vi "Lockin.AppLauncher.vi"() -> ()   [LabVIEW 2019, in "Instrument.Lockin.lvclass"]
uses:
  Instrument.Lockin.lvclass
  <vilib>/JKI/JKI SMO/SMO/Typedefs/SMOState --Enum.ctl
  <vilib>/JKI/JKI SMO/SMO.UI/Typedefs/SMO.UI State--enum.ctl
  C:/Program Files (x86)/National Instruments/LabVIEW 2019/vi.lib/JKI/JKI SMO/SMO/SMO.lvclass
  C:/Program Files (x86)/National Instruments/LabVIEW 2019/user.lib/LevyLab/Instrument Framework/SMOs/Instrument/Instrument.lvclass
  Instrument UI.Lockin/Instrument UI.Lockin.lvclass
  C:/Program Files (x86)/National Instruments/LabVIEW 2019/vi.lib/JKI/JKI SMO/SMO.UI/SMO.UI.lvclass
  C:/Program Files (x86)/National Instruments/LabVIEW 2019/user.lib/LevyLab/Instrument Framework/SMOs/Instrument UI/Instrument UI.lvclass
  <vilib>/JKI/JKI SMO/SMO/SMO.lvclass/SMO.ctl
  <vilib>/JKI/JKI SMO/SMO.UI/SMO.UI.lvclass/SMO.UI.ctl
  <vilib>/numeric/Random Number (Range) U64.vi
  <vilib>/JKI/JKI SMO/SMO/Private/ReftoDVR--SMO.vi
  <vilib>/JKI/JKI SMO/SMO.UI/SMO.UI.ReftoDVR.vi
  <vilib>/numeric/sub_Random U32.vi
  <vilib>/JKI/JKI SMO/SMO/SMO.lvclass
  <vilib>/JKI/JKI SMO/SMO.UI/SMO.UI.lvclass
  <userlib>/LevyLab/Instrument Framework/SMOs/Instrument UI/Instrument UI.lvclass
panel:
  out "error out":errorcluster
  in  "Splash Status":string="Push Start to Start..." caption="String"
  in  "Debug Mode?":bool
  in  "Start":bool=TRUE
  in  "Stop":bool=TRUE
  out "version":string
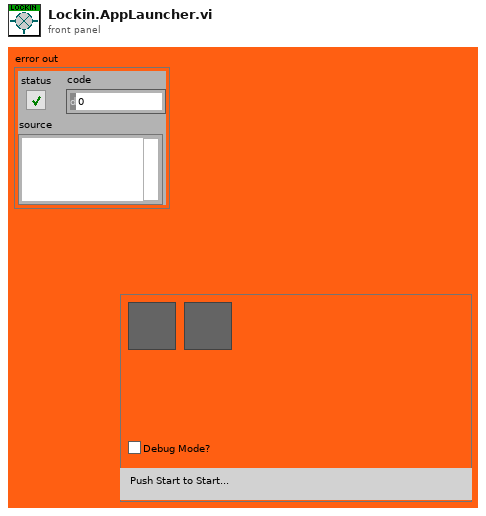
[diagram p1: front panel]
types:
  T1 = typedef "SMO.lvclass/SMOState --Enum.ctl" = enum16{"unknown", "Created", "Started", "Stopped"}
  T2 = typedef "SMO.UI.lvclass/SMO.UI State--enum.ctl" = enum16{"unknown", "Opened", "Closed"}
  T3 = enum32{"Invalid", "Standard", "Closed", "Hidden", "Minimized", "Maximized"}
  T4 = enum32{"invalid app kind", "Development System", "Run Time System", "Student Edition", "Embedded LabVIEW", "Evaluation", "Custom"}
  T5 = cluster{"Core":cluster{"Current VI Reference":refnum<vi>, "Close Panel on Exit?":bool}, "Instrument.Lockin":refnum<class "Instrument.Lockin.lvclass">, "Instrument UI.Lockin":refnum<class "Instrument UI.Lockin.lvclass">}
  T6 = cluster{"Current VI Reference":refnum<vi>, "Close Panel on Exit?":bool}
  T7 = typedef "SMO.lvclass/Public Events.ctl" = cluster{"Error":refnum<user-event>, "State":refnum<user-event>, "Reserve State":refnum<user-event>}
  T8 = typedef "SMO.UI.lvclass/PublicEvents--Cluster.ctl" = cluster{"UI Hidden":refnum<user-event>, "UI State":refnum<user-event>}
  T9 = cluster{"Event Registration Refnum":refnum<event-registration>, "Event Registration Refnum":refnum<event-registration>}
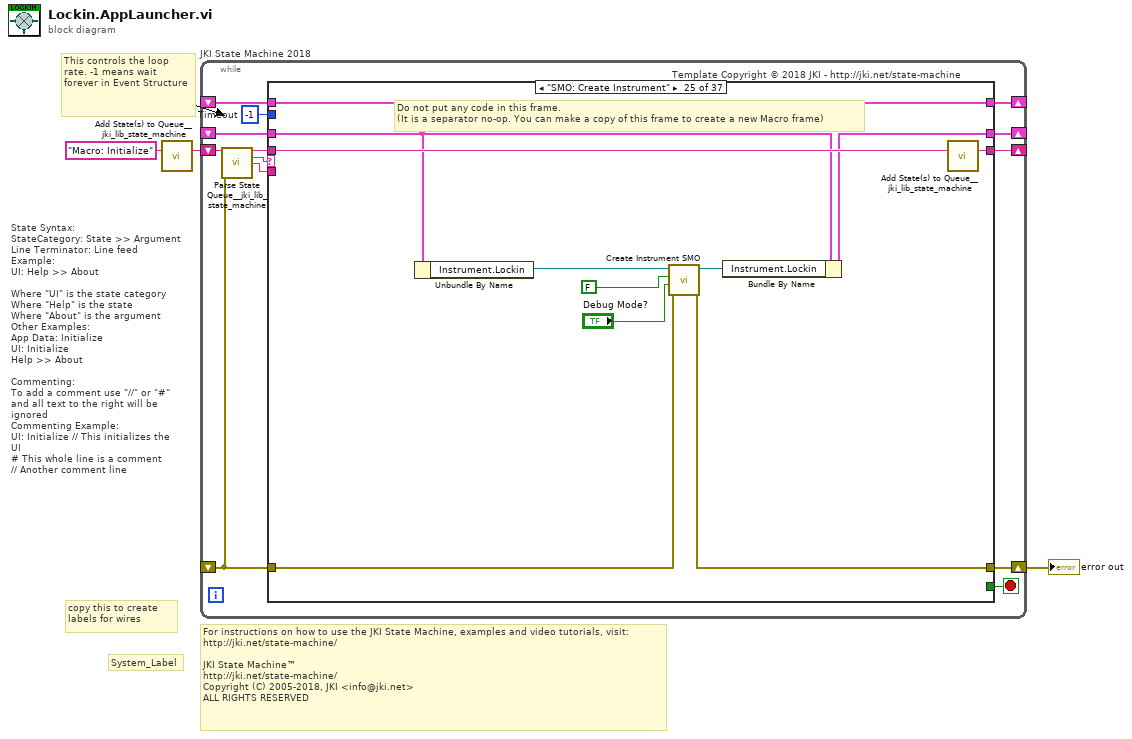
[diagram p0: block diagram]
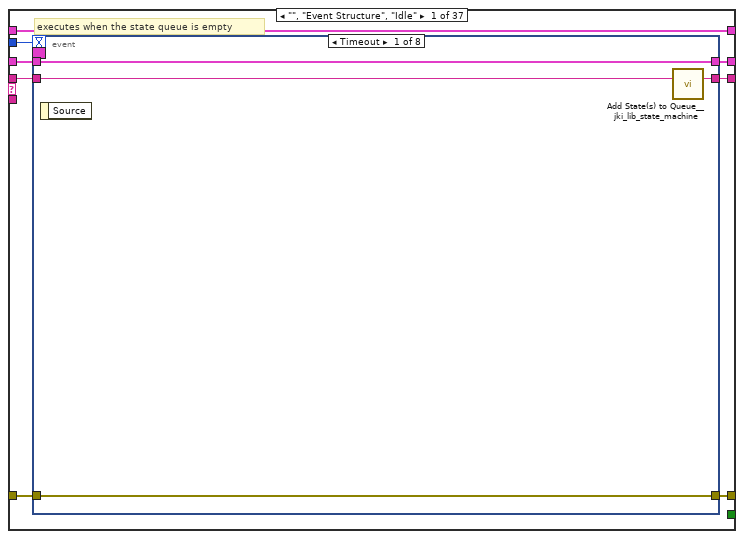
[diagram p2: hidden frame]
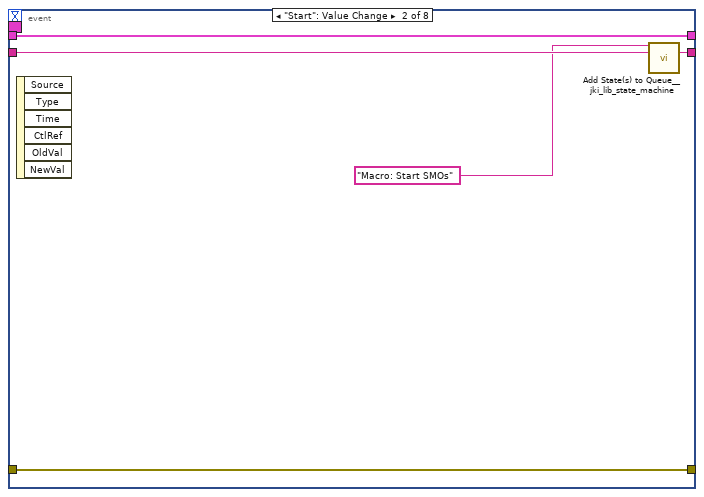
[diagram p3: hidden frame]
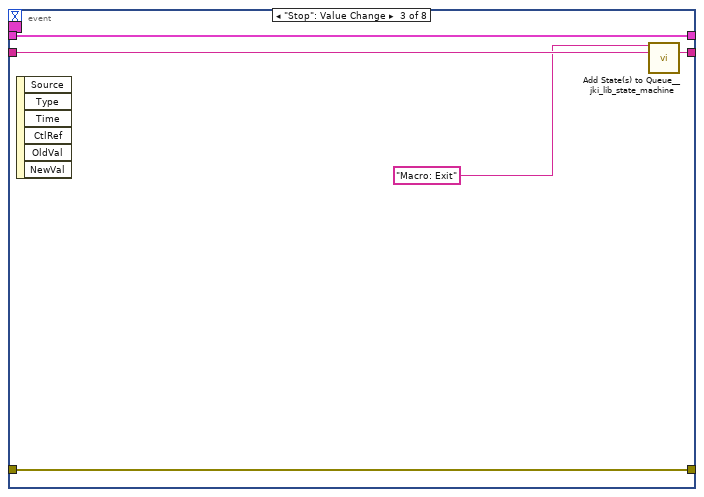
[diagram p4: hidden frame]
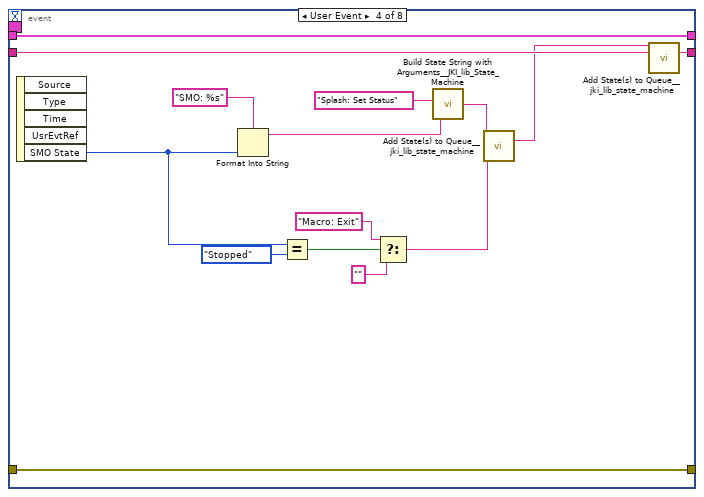
[diagram p5: hidden frame]
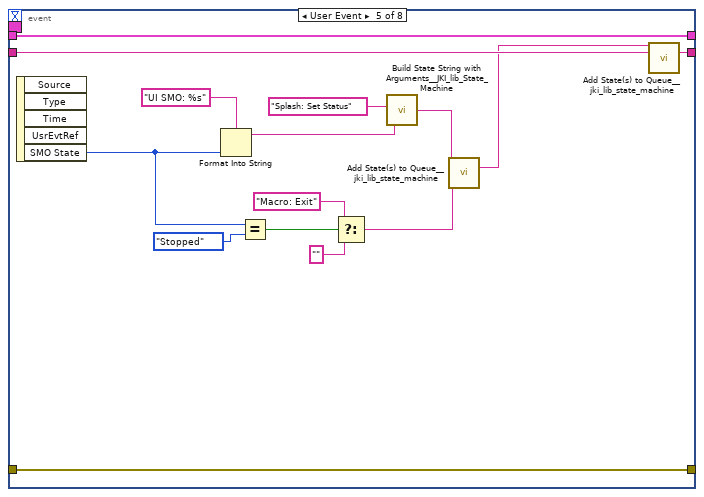
[diagram p6: hidden frame]
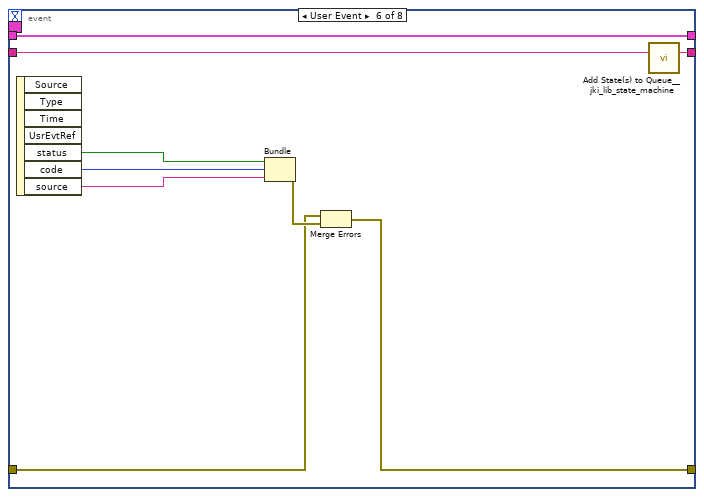
[diagram p7: hidden frame]
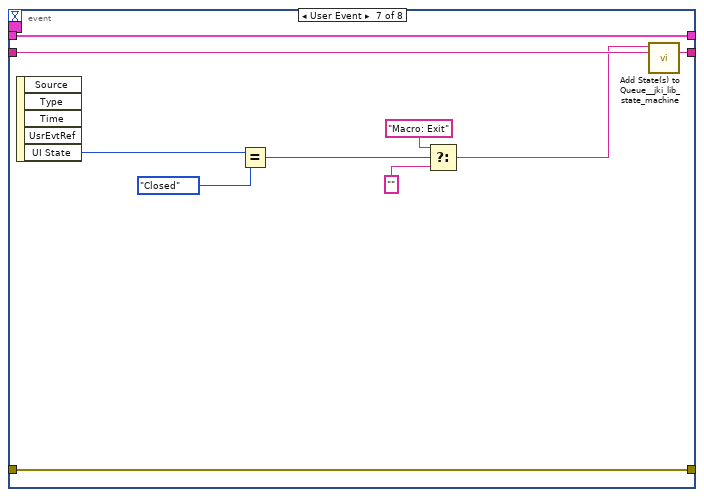
[diagram p8: hidden frame]
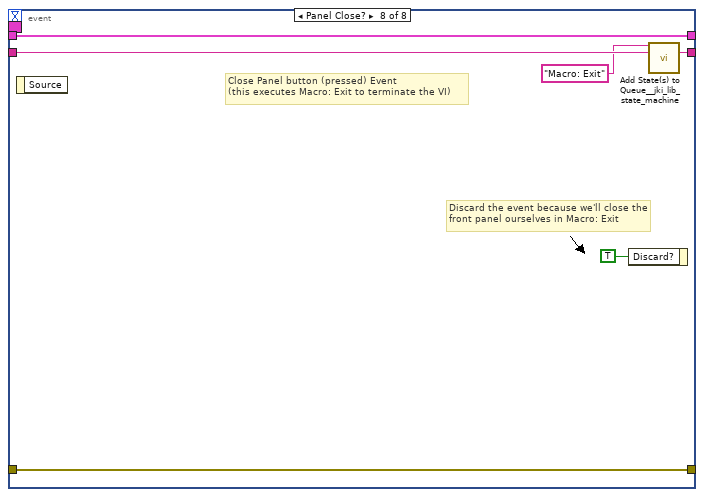
[diagram p9: hidden frame]
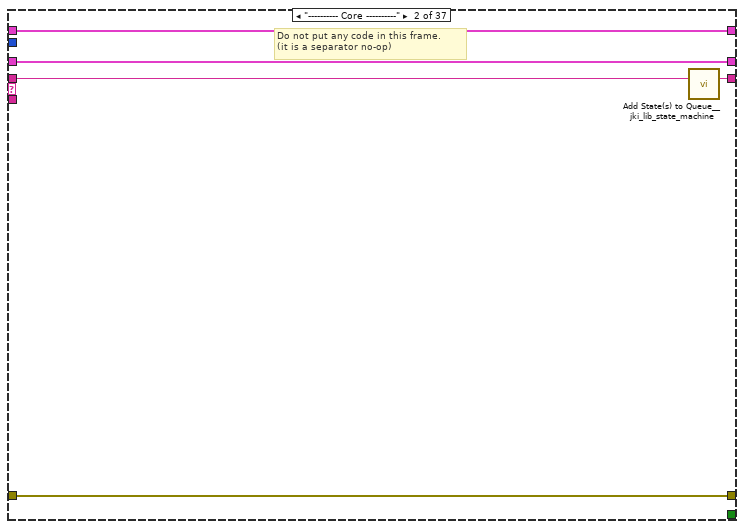
[diagram p10: hidden frame]
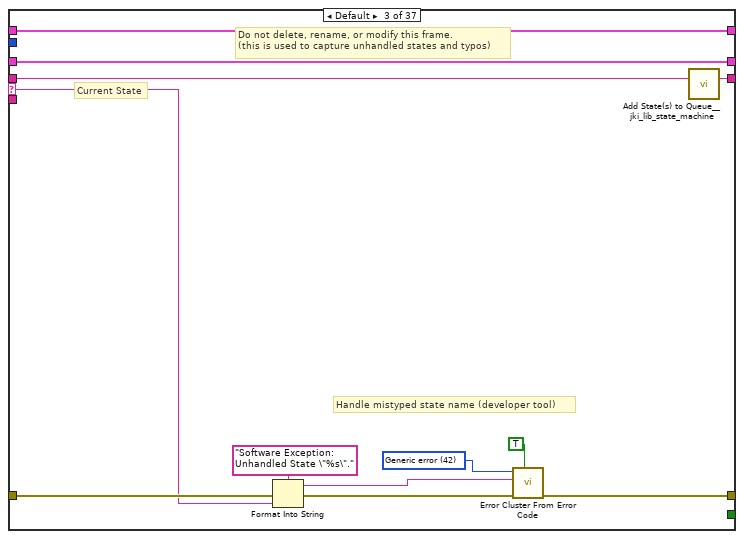
[diagram p11: hidden frame]
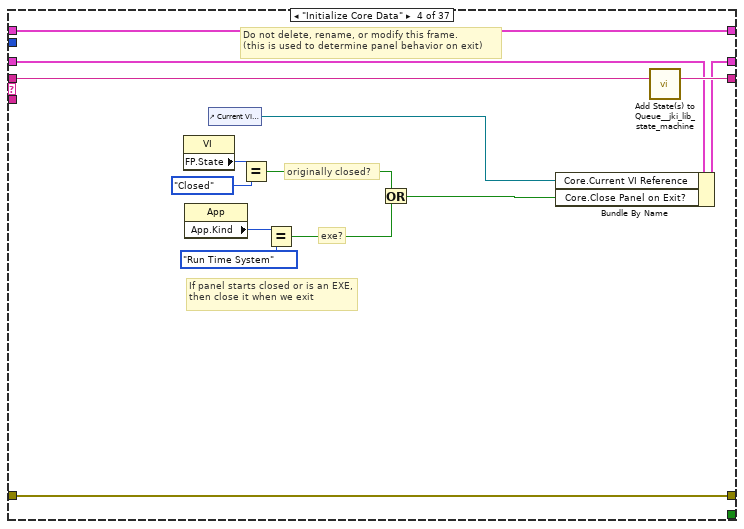
[diagram p12: hidden frame]
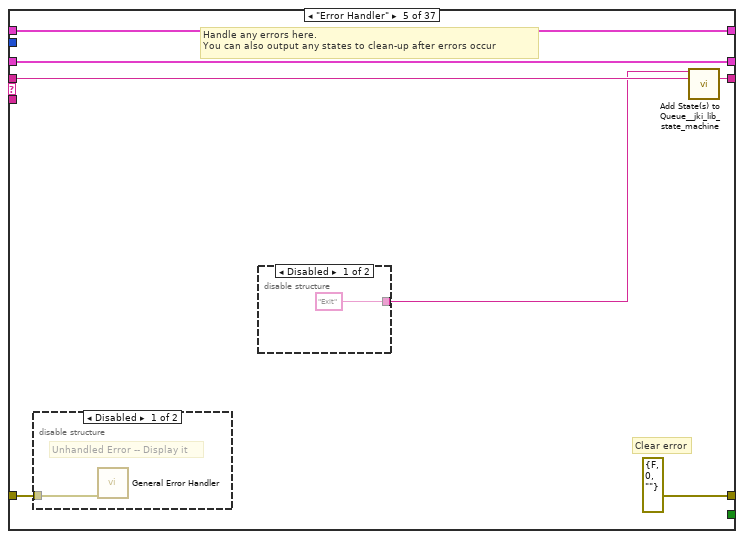
[diagram p13: hidden frame]
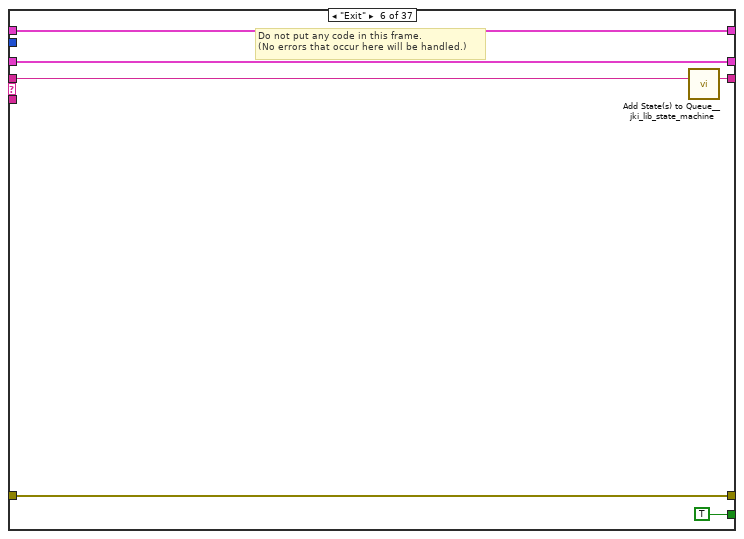
[diagram p16: hidden frame]
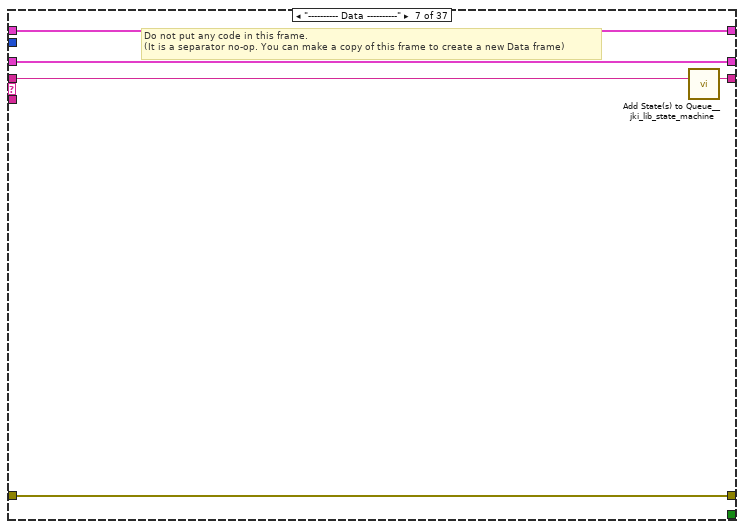
[diagram p17: hidden frame]
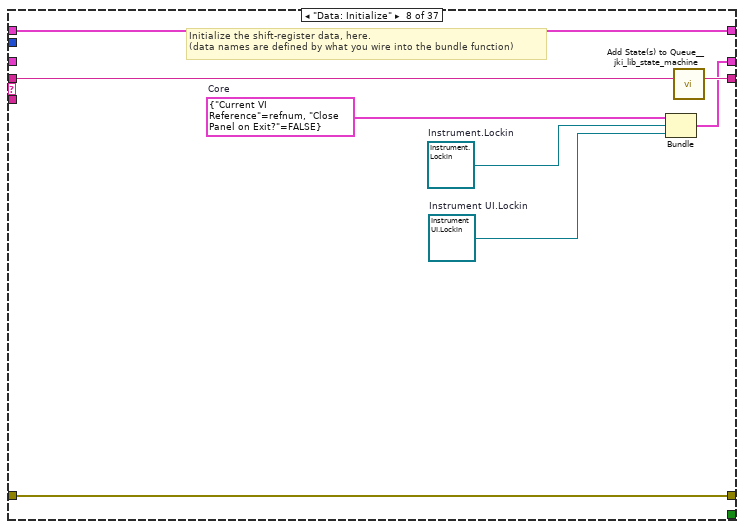
[diagram p18: hidden frame]
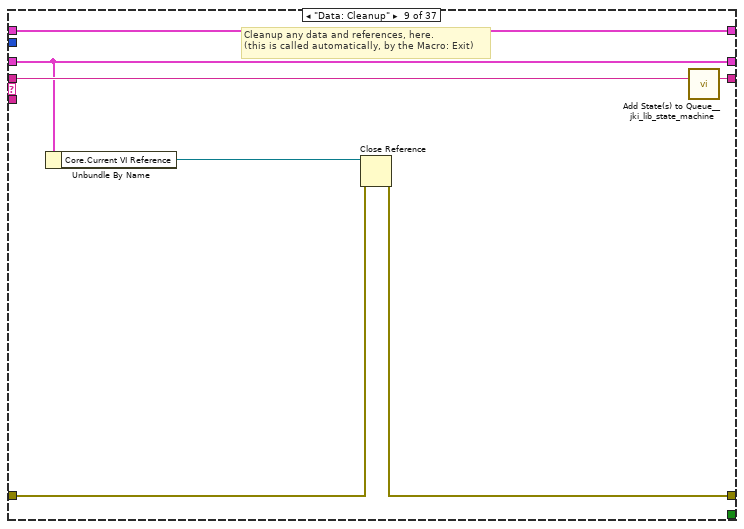
[diagram p19: hidden frame]
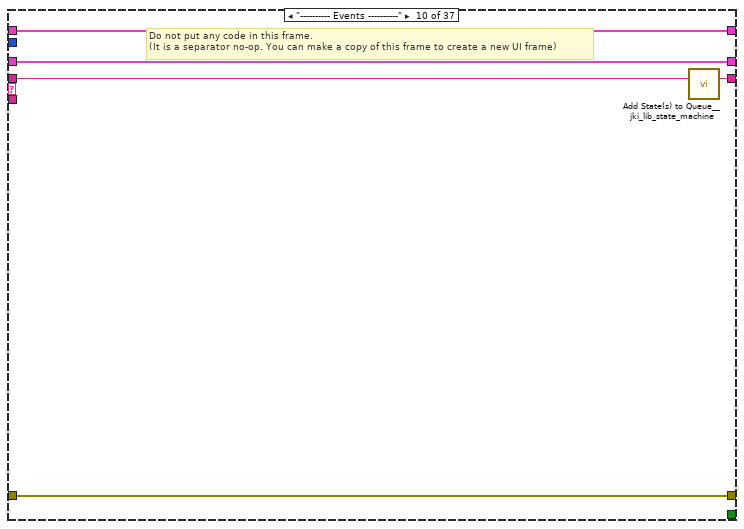
[diagram p20: hidden frame]
diagram:
  # "For instructions on how to use the JKI State Machine, examples and video tutorials, visit:\nhttp://jki.net/state-machine/\n\nJKI State Machine™\nhttp://jki.net/state-machine/\nCopyright (C) 2005-2018, JKI <info@jki.net>\nALL RIGHTS RESERVED"
  # "State Syntax:\nStateCategory: State >> Argument\nLine Terminator: Line feed\nExample:\nUI: Help >> About\n\nWhere \"UI\" is the state category\nWhere \"Help\" is the state\nWhere \"About\" is the argument\nOther Examples:\nApp Data: Initialize\nUI: Initialize\nHelp >> About\n\nCommenting:\nTo add a comment use \"//\" or \"#\" and all text to the right will be ignored\nCommenting Example:\nUI: Initialize // This initializes the UI\n# This whole line is a comment\n// Another comment line"
  # "copy this to create labels for wires"
  # "This controls the loop rate. -1 means wait forever in Event Structure"
  # "System_Label"
  n1 = call <vilib>:"Add State(s) to Queue__jki_lib_state_machine.vi"("State(s) in (\"\")"="Macro: Initialize") -> ("States Out"=w3:string)  [unwired: 14 in]
  n2 = while "JKI State Machine 2018" {
    shift-right: [w9] -> _
    shift-left: _ -> [w4]
    shift-right: [w12] -> w1
    shift-left: _ -> [w7]
    shift-right: [w11] -> _
    shift-left: w3 -> [w13]
    shift-right: [w6] -> _
    shift-left: _ -> [w5]
    stop <- w10 stop-if-true
    w8 = -1  # Timeout
    # "Template Copyright © 2018 JKI - http://jki.net/state-machine"
    n3 = call <vilib>:"Parse State Queue__jki_lib_state_machine.vi"("State Queue"=w13, "Error In (no error)"=w7) -> ("Remaining States"=w15:string, "Current State"=w16:string, "Arguments"=w14:string)  [unwired: 11 in]
    n4 = case shown="\"SMO: Create Instrument\"" w16 {
      selector: w16 -> [_ _ w100 _ _ _ _ _ _ _ _ _ _ _ _ _ _ _ _ _ _ _ _ _ _ _ _ _ _ _ _ _ _ _ _ _ _]
      tunnel: w15 -> [w24 w98 w104 w124 w131 w139 w144 w152 w159 w164 w179 w185 w190 w198 w205 w217 w298 w303 w308 w314 w320 w326 w338 w343 w354 w363 w374 w389 w403 w410 w421 w436 w451 w466 w475 w482 w487]
      tunnel: w14 -> [_ _ _ _ _ _ _ _ _ _ _ _ _ _ w200 w211 _ _ _ _ _ _ _ _ _ _ _ _ _ _ _ _ _ _ _ w479 _]
      tunnel: [w21 w96 w106 w121 errorcluster {"status"=FALSE, "code"=0, "source"=""} ("error out") w136 w142 w149 w155 w162 w168 w180 w188 w193 w201 w214 w289 w301 w306 w312 w318 w324 w336 w341 w347 w355 w371 w385 w397 w404 w417 w432 w448 w463 w473 w477 w485] -> w12
      tunnel: w7 -> [w20 w96 w105 w121 w127 w136 w142 w149 w156 w162 w170 w181 w188 w195 w202 w215 w290 w301 w306 w312 w318 w324 w336 w341 w344 w356 w369 w381 w396 w405 w414 w429 w446 w459 w473 w478 w485]
      tunnel: [w23 w97 w103 w123 w130 w138 w143 w151 w158 w163 w178 w184 w189 w197 w204 w216 w297 w302 w307 w313 w319 w325 w337 w342 w353 w362 w373 w388 w402 w409 w420 w435 w450 w465 w474 w481 w486] -> w11
      tunnel: [_ _ _ _ _ TRUE _ _ _ _ _ _ _ _ _ _ _ _ _ _ _ _ _ _ _ _ _ _ _ _ _ _ _ _ _ _ _] -> w10
      tunnel: [w19 w95 w102 w122 w128 w137 w141 w150 w153 w161 w173 w183 w187 w196 w203 w213 w287 w300 w305 w311 w317 w323 w335 w340 w351 w358 w370 w386 w399 w407 w418 w433 w447 w462 w472 w480 w484] -> w9
      tunnel: w8 -> [w18 _ _ _ _ _ _ _ _ _ _ _ _ _ _ _ _ _ _ _ _ _ _ _ _ _ _ _ _ _ _ _ _ _ _ _ _]
      tunnel: [w17 w94 w99 w111 w125 w134 w140 w147 w154 w160 w176 w182 w186 w194 w199 w210 w288 w299 w304 w309 w316 w322 w329 w339 w352 w361 w372 w387 w401 w408 w419 w434 w449 w464 w471 w476 w483] -> w6
      tunnel: w5 -> [w17 w94 w99 w111 w125 w134 w140 w147 w154 w160 _ w182 w186 w194 w199 w210 w288 w299 w304 w309 w316 w322 w329 w339 w352 w361 w372 w387 w401 w408 w419 w434 w449 w464 w471 w476 w483]
      tunnel: w4 -> [w22 w95 w102 w117 w128 w137 w141 _ w153 w161 w173 w183 w187 w196 w203 w213 w287 w300 w305 w311 w317 w323 w335 w340 w346 w359 w370 w386 w400 w407 w418 w433 w447 w462 w472 w480 w484]
      frame "", "Event Structure", "Idle" {
        # "executes when the state queue is empty"
        n5 = event shown="[0] Timeout" {
          selector: w17 -> [_ _ _ _ _ _ _ _]
          dyn-events: _ -> [_ _ _ _ _ _ _ _]
          timeout: w18 -> [_ _ _ _ _ _ _ _]
          tunnel: w24 -> [w28 w33 w38 w53 w68 w77 w87 w93]
          tunnel: [w27 w32 w37 w52 w67 w76 w86 w92] -> w23
          tunnel: w22 -> [w25 w30 w35 w50 w65 w75 w85 w90]
          tunnel: [w26 w31 w36 w51 w66 w72 w84 w91] -> w21
          tunnel: w20 -> [w26 w31 w36 w51 w66 w73 w84 w91]
          tunnel: [w25 w30 w35 w50 w65 w75 w85 w90] -> w19
          event Timeout {
            n6 = event-data() -> ()  [unwired: 1 in, 1 out]
            n7 = call <vilib>:"Add State(s) to Queue__jki_lib_state_machine.vi"("State(s) in (\"\")"=w28) -> ("States Out"=w27:string)  [unwired: 14 in]
          }
          event "Start": Value Change {
            n8 = event-data() -> ()  [unwired: 1 in, 6 out]
            n9 = call <vilib>:"Add State(s) to Queue__jki_lib_state_machine.vi"("State(s) in Front (\"\")"="Macro: Start SMOs" ("State(s) in Front (\"\")"), "State(s) in (\"\")"=w33) -> ("States Out"=w32:string)  [unwired: 13 in]
          }
          event "Stop": Value Change {
            n10 = event-data() -> ()  [unwired: 1 in, 6 out]
            n11 = call <vilib>:"Add State(s) to Queue__jki_lib_state_machine.vi"("State(s) in Front (\"\")"="Macro: Exit" ("State(s) in Front (\"\")"), "State(s) in (\"\")"=w38) -> ("States Out"=w37:string)  [unwired: 13 in]
          }
          event User Event {
            n12 = event-data() -> ("SMO State"=w45:T1)  [unwired: 1 in, 4 out]
            n13 = Format Into String(format string="SMO: %s", w45) -> (resulting string=w42:string)  [unwired: 2 in, 1 out]
            n14 = Equal?(x=w45, y=SMOState_--Enum."Stopped") -> (x = y?=w48:bool)
            n15 = Select(t="Macro: Exit", s=w48, f="" ("State(s) in Front (\"\")")) -> (s? t:f=w40:string)
            n16 = call <vilib>:"Build State String with Arguments__JKI_lib_State_Machine.vi"("Arguments (\"\")"=w42, "State"="Splash: Set Status" ("t")) -> ("State with Arguments"=w41:string)  [unwired: 4 in]
            n17 = call <vilib>:"Add State(s) to Queue__jki_lib_state_machine.vi"("State(s) in Front (\"\")"=w41, "State(s) at Back (\"\")"=w40) -> ("States Out"=w39:string)  [unwired: 13 in]
            n18 = call <vilib>:"Add State(s) to Queue__jki_lib_state_machine.vi"("State(s) in Front (\"\")"=w39, "State(s) in (\"\")"=w53) -> ("States Out"=w52:string)  [unwired: 13 in]
          }
          event User Event {
            n19 = event-data() -> ("SMO State"=w56:T1)  [unwired: 1 in, 4 out]
            n20 = Format Into String(format string="UI SMO: %s", w56) -> (resulting string=w60:string)  [unwired: 2 in, 1 out]
            n21 = Equal?(x=w56, y=SMOState_--Enum."Stopped") -> (x = y?=w64:bool)
            n22 = Select(t="Macro: Exit", s=w64, f="" ("State(s) in Front (\"\")")) -> (s? t:f=w59:string)
            n23 = call <vilib>:"Build State String with Arguments__JKI_lib_State_Machine.vi"("Arguments (\"\")"=w60, "State"="Splash: Set Status" ("t")) -> ("State with Arguments"=w57:string)  [unwired: 4 in]
            n24 = call <vilib>:"Add State(s) to Queue__jki_lib_state_machine.vi"("State(s) in Front (\"\")"=w57, "State(s) at Back (\"\")"=w59) -> ("States Out"=w58:string)  [unwired: 13 in]
            n25 = call <vilib>:"Add State(s) to Queue__jki_lib_state_machine.vi"("State(s) in Front (\"\")"=w58, "State(s) in (\"\")"=w68) -> ("States Out"=w67:string)  [unwired: 13 in]
          }
          event User Event {
            n26 = event-data() -> ("status"=w69:bool, "code"=w71:i32, "source"=w70:string)  [unwired: 1 in, 4 out]
            n27 = Bundle("status"=w69, "code"=w71, "source"=w70) -> (w74:errorcluster)  [unwired: 1 in]
            n28 = Merge Errors(w73, w74) -> (w72:errorcluster)
            n29 = call <vilib>:"Add State(s) to Queue__jki_lib_state_machine.vi"("State(s) in (\"\")"=w77) -> ("States Out"=w76:string)  [unwired: 14 in]
          }
          event User Event {
            n30 = event-data() -> ("UI State"=w83:T2)  [unwired: 1 in, 4 out]
            n31 = Equal?(x=w83, y=SMO.UI_State--enum."Closed" ("UI State")) -> (x = y?=w81:bool)
            n32 = Select(t="Macro: Exit", s=w81, f="") -> (s? t:f=w78:string)
            n33 = call <vilib>:"Add State(s) to Queue__jki_lib_state_machine.vi"("State(s) in Front (\"\")"=w78, "State(s) in (\"\")"=w87) -> ("States Out"=w86:string)  [unwired: 13 in]
          }
          event Panel Close? {
            # "Discard the event because we'll close the front panel ourselves in Macro: Exit"
            # "Close Panel button (pressed) Event\n(this executes Macro: Exit to terminate the VI)"
            n34 = event-data() -> ()  [unwired: 1 in, 1 out]
            n35 = event-data("Discard?"=TRUE) -> ()  [unwired: 1 in, 1 out]
            n36 = call <vilib>:"Add State(s) to Queue__jki_lib_state_machine.vi"("State(s) in Front (\"\")"="Macro: Exit", "State(s) in (\"\")"=w93) -> ("States Out"=w92:string)  [unwired: 13 in]
          }
        }
      }
      frame "---------- Core ----------" {
        # "Do not put any code in this frame.\n(it is a separator no-op)"
        n37 = call <vilib>:"Add State(s) to Queue__jki_lib_state_machine.vi"("State(s) in (\"\")"=w98) -> ("States Out"=w97:string)  [unwired: 14 in]
      }
      frame Default {
        w109 = 42 items=["No error", "Argument error", "Memory is full", "Out of zone", "End of file", "File already open", "Generic file I/O error", "File not found", "File permission error", "Disk is full", "Duplicate path", "Too many files open", "System feature not enabled", "Resource file not found", "Cannot add resource", "Resource not found", "Image not found", "Image memory error", "Pen does not exist", "Config type invalid", "Config token not found", "Config parse error", "Config memory error", "Bad external code format", "Bad external code offset", "External code not present", "Null window", "Destroy window error", "Null menu", "Print aborted", "Bad print record", "Print driver error", "Windows error during printing", "Memory error during printing", "Print dialog error", "Generic print error", "Invalid device refnum", "Device not found", "Device parameter error", "Device unit error", "Cannot open device", "Device call aborted", "Generic error", "Cancelled by user", "Object ID too low", "Object ID too high", "Object not in heap", "Unknown heap", "Unknown object (invalid DefProc)", "Unknown object (DefProc not in table)", "Message out of range", "Invalid (null) method", "Unknown message", "Manager call not supported", "Bad address", "Network operation in progress", "Network operation timed out", "Connection is busy", "Network attribute not supported", "Network error", "Address in use", "System out of memory", "Connection aborted", "Connection refused", "Not connected", "Already connected", "Connection closed", "Initialization error (interapplication manager)", "Bad occurrence", "Wait on unbound occurrence handler", "Occurrence queue overflow", "Datalog type conflict", "Unused", "Unrecognized type (interapplication manager)", "Memory corrupt", "Failed to make temporary DLL", "Old CIN version", "Drag socket not found", "Failed to load drop-object", "Failed to register OLE object", "Failed to release OLE object", "Format specifier type mismatch", "Unknown format specifier", "Too few format specifiers", "Too many format specifiers", "Scan failed", "Newer CIN version", "Error converting to variant", "Runtime menu error", "Password tampered", "Variant attribute not found", "Incompatible variant data type", "Event data is not available", "Event Store is not present", "Occurrence is not found", "Event Queue is not created", "Event info is not available", "Refnum passed is NULL", "Error retrieving Class GUID", "Error retrieving CoClass GUID", "Error retrieving TypeLib GUID.", "Bad built application magic bytes.", "Specific driver is different from the specific driver associated with the Logical Name.", "There is no session opened to the class driver.", "Max Error", "MAX - Error with config objects", "MAX - Error loading configuration", "MAX - Group not supported"]
        # "Current State"
        # "Do not delete, rename, or modify this frame.\n(this is used to capture unhandled states and typos)"
        # "Handle mistyped state name (developer tool)"
        n38 = Format Into String(format string="Software Exception: Unhandled State \"%s\"." ("message"), error in=w105, w100) -> (resulting string=w108:string, error out=w107:errorcluster)  [unwired: 1 in]
        n39 = call <vilib>:"Error Cluster From Error Code.vi"("show call chain? (False)"=TRUE, "error in (no error)"=w107, "error message (\"\")"=w108, "error code (0)"=w109) -> ("error out"=w106:errorcluster)  [unwired: 5 in]
        n40 = call <vilib>:"Add State(s) to Queue__jki_lib_state_machine.vi"("State(s) in (\"\")"=w104) -> ("States Out"=w103:string)  [unwired: 14 in]
      }
      frame "Initialize Core Data" {
        # "Do not delete, rename, or modify this frame.\n(this is used to determine panel behavior on exit)"
        # "originally closed?"
        # "exe?"
        # "If panel starts closed or is an EXE, then close it when we exit"
        n41 = property class="VI"() -> ("FP.State"=w114:T3)  [unwired: 2 in, 2 out]
        n42 = property class="App"() -> ("App.Kind"=w120:T4)  [unwired: 2 in, 2 out]
        n43 = control-ref of="Current VI Reference"() -> (w115:refnum<vi>)
        n44 = Equal?(x=w114, y=T3."Closed" ("Front Panel Window:State")) -> (x = y?=w112:bool)
        n45 = Equal?(x=w120, y=T4."Run Time System" ("Application:Kind")) -> (x = y?=w118:bool)
        n46 = Or(x=w112, y=w118) -> (x .or. y?=w116:bool)
        n47 = Bundle By Name(cluster=w117, "Core.Current VI Reference"=w115, "Core.Close Panel on Exit?"=w116) -> (w122:T5)
        n48 = call <vilib>:"Add State(s) to Queue__jki_lib_state_machine.vi"("State(s) in (\"\")"=w124) -> ("States Out"=w123:string)  [unwired: 14 in]
      }
      frame "Error Handler" {
        # "Handle any errors here.\nYou can also output any states to clean-up after errors occur"
        # "Clear error"
        n49 = disable-structure shown="Disabled" {
          disable-tunnel: w127 -> [w133 _]
          frame Disabled {
            # "Unhandled Error -- Display it"
            n50 = call <vilib>:"General Error Handler.vi"("error in (no error)"=w133) -> ()  [unwired: 10 in, 5 out]
          }
          frame Enabled {
          }
        }
        n51 = disable-structure shown="Disabled" {
          disable-tunnel: ["Exit" _] -> w126
          frame Disabled {
          }
          frame Enabled {
          }
        }
        n52 = call <vilib>:"Add State(s) to Queue__jki_lib_state_machine.vi"("State(s) in Front (\"\")"=w126, "State(s) in (\"\")"=w131) -> ("States Out"=w130:string)  [unwired: 13 in]
      }
      frame "Exit" {
        # "Do not put any code in this frame.\n(No errors that occur here will be handled.)"
        n53 = call <vilib>:"Add State(s) to Queue__jki_lib_state_machine.vi"("State(s) in (\"\")"=w139) -> ("States Out"=w138:string)  [unwired: 14 in]
      }
      frame "---------- Data ----------" {
        # "Do not put any code in this frame.\n(It is a separator no-op. You can make a copy of this frame to create a new Data frame)"
        n54 = call <vilib>:"Add State(s) to Queue__jki_lib_state_machine.vi"("State(s) in (\"\")"=w144) -> ("States Out"=w143:string)  [unwired: 14 in]
      }
      frame "Data: Initialize" {
        w146 = refnum<class "Instrument UI.Lockin.lvclass"> refnum  # Instrument UI.Lockin
        w145 = refnum<class "Instrument.Lockin.lvclass"> refnum  # Instrument.Lockin
        w148 = T6 {"Current VI Reference"=refnum, "Close Panel on Exit?"=FALSE}  # Core
        # "Initialize the shift-register data, here.\n(data names are defined by what you wire into the bundle function)"
        n55 = Bundle("Core"=w148, "Instrument.Lockin"=w145, "Instrument UI.Lockin"=w146) -> (w150:T5)  [unwired: 1 in]
        n56 = call <vilib>:"Add State(s) to Queue__jki_lib_state_machine.vi"("State(s) in (\"\")"=w152) -> ("States Out"=w151:string)  [unwired: 14 in]
      }
      frame "Data: Cleanup" {
        # "Cleanup any data and references, here.\n(this is called automatically, by the Macro: Exit)"
        n57 = Unbundle By Name(w153) -> ("Core.Current VI Reference"=w157:refnum<vi>)
        n58 = Close Reference(reference=w157, error in (no error)=w156) -> (error out=w155:errorcluster)
        n59 = call <vilib>:"Add State(s) to Queue__jki_lib_state_machine.vi"("State(s) in (\"\")"=w159) -> ("States Out"=w158:string)  [unwired: 14 in]
      }
      frame "---------- Events ----------" {
        # "Do not put any code in this frame.\n(It is a separator no-op. You can make a copy of this frame to create a new UI frame)"
        n60 = call <vilib>:"Add State(s) to Queue__jki_lib_state_machine.vi"("State(s) in (\"\")"=w164) -> ("States Out"=w163:string)  [unwired: 14 in]
      }
      frame "Events: Register" {
        # "Do not put any code in this frame.\n(It is a separator no-op. You can make a copy of this frame to create a new UI frame)"
        n61 = Unbundle By Name(w173) -> ("Instrument.Lockin"=w172:refnum<class "Instrument.Lockin.lvclass">, "Instrument UI.Lockin"=w171:refnum<class "Instrument UI.Lockin.lvclass">)
        n62 = call <vilib>:"GetPublicEvents.vi"("error in (no error)"=w170, "SMO"=w172) -> ("error out"=w169:errorcluster, "Public Events"=w174:T7)  [unwired: 7 in, 1 out]
        n63 = call <vilib>:"GetPublicEvents.vi"("error in (no error)"=w169, "SMO"=w171) -> ("error out"=w168:errorcluster, "Public Events"=w175:T7, "SMO out"=w166:refnum<class "Instrument UI.Lockin.lvclass">)  [unwired: 7 in]
        n64 = register-events(w174) -> (reference out=w177:refnum<event-registration>)  [unwired: 2 in, 1 out]
        n65 = call <vilib>:"SMO.UI.GetPublicEvents.vi"("SMO.UI"=w166) -> ("SMO.UI Public Events"=w165:T8)  [unwired: 8 in, 2 out]
        n66 = register-events(w175, w165) -> (reference out=w167:refnum<event-registration>)  [unwired: 2 in, 1 out]
        n67 = Bundle("Event Registration Refnum"=w177, "Event Registration Refnum"=w167) -> (w176:T9)  [unwired: 1 in]
        n68 = call <vilib>:"Add State(s) to Queue__jki_lib_state_machine.vi"("State(s) in (\"\")"=w179) -> ("States Out"=w178:string)  [unwired: 14 in]
      }
      frame "Events: Unregister" {
        # "Do not put any code in this frame.\n(It is a separator no-op. You can make a copy of this frame to create a new UI frame)"
        n69 = Unregister For Events(event registration refnum=w182, error in=w181) -> (error out=w180:errorcluster)
        n70 = call <vilib>:"Add State(s) to Queue__jki_lib_state_machine.vi"("State(s) in (\"\")"=w185) -> ("States Out"=w184:string)  [unwired: 14 in]
      }
      frame "---------- UI ----------" {
        # "Do not put any code in this frame.\n(It is a separator no-op. You can make a copy of this frame to create a new UI frame)"
        n71 = call <vilib>:"Add State(s) to Queue__jki_lib_state_machine.vi"("State(s) in (\"\")"=w190) -> ("States Out"=w189:string)  [unwired: 14 in]
      }
      frame "UI: Initialize" {
        # "Initialize the User Interface, here.\n(this is called automatically, by the Macro: Init)"
        n72 = invoke on="Start" class="Bool (strict)" method="Reinit To Default"() -> ()  [unwired: 3 in, 3 out]
        n73 = invoke on="Stop" class="Bool (strict)" method="Reinit To Default"() -> ()  [unwired: 3 in, 3 out]
        n74 = invoke on="error out" class="Clust (strict)" method="Reinit To Default"() -> ()  [unwired: 3 in, 3 out]
        n75 = call <userlib>:"Fit VI window to Largest Dec__ogtk.vi"("error in (no error)"=w195, "border spacing (2 px)"=-1) -> ("error out"=w193:errorcluster)  [unwired: 4 in, 1 out]
        n76 = call <userlib>:"MGI Get Executable Version.vi"() -> ("Version"=→"version":string)  [unwired: 7 in]
        n77 = call <vilib>:"Add State(s) to Queue__jki_lib_state_machine.vi"("State(s) in (\"\")"=w198) -> ("States Out"=w197:string)  [unwired: 14 in]
      }
      frame "UI: Cursor Set" {
        # "Argument"
        # "Set and Unset Cursor Busy.\n(Usage: \"UI: Cursor Set >> Busy|Idle\")"
        n78 = case shown="\"Busy\"" w200 {
          tunnel: w202 -> [w207 w209]
          tunnel: [w206 w208] -> w201
          frame "Idle", Default {
            n79 = call <vilib>:"Unset Busy.vi"("error in (no error)"=w207) -> ("error out"=w206:errorcluster)  [unwired: 10 in]
          }
          frame "Busy" {
            n80 = call <vilib>:"Set Busy.vi"("error in (no error)"=w209) -> ("error out"=w208:errorcluster)  [unwired: 9 in, 1 out]
          }
        }
        n81 = call <vilib>:"Add State(s) to Queue__jki_lib_state_machine.vi"("State(s) in (\"\")"=w205) -> ("States Out"=w204:string)  [unwired: 14 in]
      }
      frame "UI: Front Panel State" {
        # "Argument"
        # "Set Front Panel Open or Closed\n(Usage: \"UI: Front Panel State >> Open|Close\")"
        n82 = Unbundle By Name(w213) -> ("Core.Current VI Reference"=w212:refnum<vi>)
        n83 = case shown="\"Open\", \"Standard\", Default" w211 {
          tunnel: w215 -> [w223 w238 w249 w262 w275]
          tunnel: [w225 w239 w251 w264 w277] -> w214
          tunnel: w212 -> [w224 w236 w250 w263 w276]
          frame "Open", "Standard", Default {
            w218 = T3."Standard" ("State")
            n84 = property class="VI"(reference=w224, error in=w223) -> (reference out=w221:refnum<vi>, error out=w222:errorcluster, "FP.State"=w220:T3)
            n85 = Not Equal?(x=w220, y=w218) -> (x != y?=w219:bool)
            n86 = case shown="False" w219 {
              tunnel: [w229 w231] -> w225
              tunnel: w222 -> [w228 w231]
              tunnel: w221 -> [w227 _]
              tunnel: w218 -> [w226 _]
              frame True {
                n87 = invoke class="VI" method="FP.Open"(reference=w227, error in=w228, "Activate"=TRUE, "State"=w226) -> (error out=w229:errorcluster)  [unwired: 1 in, 4 out]
              }
              frame False {
              }
            }
          }
          frame "Close", "Closed" {
            n88 = property class="VI"(reference=w236, error in=w238) -> (reference out=w235:refnum<vi>, error out=w237:errorcluster, "FP.State"=w233:T3)
            n89 = Not Equal?(x=w233, y=T3."Closed" ("Front Panel Window:State")) -> (x != y?=w232:bool)
            n90 = case shown="True" w232 {
              tunnel: [w240 w243] -> w239
              tunnel: w237 -> [w240 w242]
              tunnel: w235 -> [_ w241]
              frame False {
              }
              frame True {
                n91 = invoke class="VI" method="FP.Close"(reference=w241, error in=w242) -> (error out=w243:errorcluster)  [unwired: 1 in, 2 out]
              }
            }
          }
          frame "Hidden", "Hide" {
            w244 = T3."Hidden" ("State")
            n92 = property class="VI"(reference=w250, error in=w249) -> (reference out=w247:refnum<vi>, error out=w248:errorcluster, "FP.State"=w246:T3)
            n93 = Not Equal?(x=w246, y=w244) -> (x != y?=w245:bool)
            n94 = case shown="True" w245 {
              tunnel: [w255 w256] -> w251
              tunnel: w248 -> [w254 w256]
              tunnel: w247 -> [w253 _]
              tunnel: w244 -> [w252 _]
              frame True {
                n95 = invoke class="VI" method="FP.Open"(reference=w253, error in=w254, "State"=w252) -> (error out=w255:errorcluster)  [unwired: 2 in, 4 out]
              }
              frame False {
              }
            }
          }
          frame "Minimize", "Minimized" {
            w257 = T3."Minimized" ("State")
            n96 = property class="VI"(reference=w263, error in=w262) -> (reference out=w260:refnum<vi>, error out=w261:errorcluster, "FP.State"=w259:T3)
            n97 = Not Equal?(x=w259, y=w257) -> (x != y?=w258:bool)
            n98 = case shown="True" w258 {
              tunnel: [w268 w269] -> w264
              tunnel: w261 -> [w267 w269]
              tunnel: w260 -> [w266 _]
              tunnel: w257 -> [w265 _]
              frame True {
                n99 = invoke class="VI" method="FP.Open"(reference=w266, error in=w267, "State"=w265) -> (error out=w268:errorcluster)  [unwired: 2 in, 4 out]
              }
              frame False {
              }
            }
          }
          frame "Maximize", "Maximized" {
            w270 = T3."Maximized" ("State")
            n100 = property class="VI"(reference=w276, error in=w275) -> (reference out=w273:refnum<vi>, error out=w274:errorcluster, "FP.State"=w272:T3)
            n101 = Not Equal?(x=w272, y=w270) -> (x != y?=w271:bool)
            n102 = case shown="True" w271 {
              tunnel: [w281 w282] -> w277
              tunnel: w274 -> [w280 w282]
              tunnel: w273 -> [w279 _]
              tunnel: w270 -> [w278 _]
              frame True {
                n103 = invoke class="VI" method="FP.Open"(reference=w279, error in=w280, "State"=w278) -> (error out=w281:errorcluster)  [unwired: 2 in, 4 out]
              }
              frame False {
              }
            }
          }
        }
        n104 = call <vilib>:"Add State(s) to Queue__jki_lib_state_machine.vi"("State(s) in (\"\")"=w217) -> ("States Out"=w216:string)  [unwired: 14 in]
      }
      frame "UI: Set Background Color" {
        # "Do not put any code in this frame.\n(It is a separator no-op. You can make a copy of this frame to create a new UI frame)"
        n105 = property class="VI"(error in=w290) -> (error out=w292:errorcluster, "Panel"=w293:refnum<vi>)  [unwired: 1 in, 1 out]
        n106 = property class="Pnl"(reference=w293, error in=w292) -> (error out=w291:errorcluster, "Panes[]"=w294:refnum<vi>[])  [unwired: 1 out]
        n107 = call-poly <vilib>:"Random Number (Range).vi"("lower bound (0)"=u32 16736018 ("Color Box"), "upper bound (100)"=u32 16711708 ("Color Box")) -> ("number"=w284:u64)  [unwired: 9 in]
        n108 = Index Array(array=w294, index=0) -> (element=w296:refnum<vi>)
        n109 = To Unsigned Long Integer(number=w284) -> (unsigned 32bit integer=w283:u32)
        n110 = property class="Pane"(reference=w296, error in=w291, "PaneColor"=w283) -> (error out=w289:errorcluster)  [unwired: 1 out]
        n111 = call <vilib>:"Add State(s) to Queue__jki_lib_state_machine.vi"("State(s) in (\"\")"=w298) -> ("States Out"=w297:string)  [unwired: 14 in]
      }
      frame "UI: Exit" {
        # "Do not put any code in this frame.\n(It is a separator no-op. You can make a copy of this frame to create a new UI frame)"
        n112 = invoke on="Start" class="Bool (strict)" method="Reinit To Default"() -> ()  [unwired: 3 in, 3 out]
        n113 = invoke on="Stop" class="Bool (strict)" method="Reinit To Default"() -> ()  [unwired: 3 in, 3 out]
        n114 = call <vilib>:"Add State(s) to Queue__jki_lib_state_machine.vi"("State(s) in (\"\")"=w303) -> ("States Out"=w302:string)  [unwired: 14 in]
      }
      frame "---------- Macro ----------" {
        # "Do not put any code in this frame.\n(It is a separator no-op. You can make a copy of this frame to create a new Macro frame)"
        n115 = call <vilib>:"Add State(s) to Queue__jki_lib_state_machine.vi"("State(s) in (\"\")"=w308) -> ("States Out"=w307:string)  [unwired: 14 in]
      }
      frame "Macro: Initialize" {
        # "Initialization Macro\n(This is called once, when the VI starts)"
        n116 = call <vilib>:"Add State(s) to Queue__jki_lib_state_machine.vi"("State(s) in Front (\"\")"="Data: Initialize\nInitialize Core Data\n//Events: Register\nUI: Initialize\nUI: Front Panel State >> Open\nUI: Set Background Color\nSplash: Set Status >> Push Start to Start...", "State(s) in (\"\")"=w314) -> ("States Out"=w313:string)  [unwired: 13 in]
      }
      frame "Macro: Start SMOs" {
        # "Do not put any code in this frame.\n(It is a separator no-op. You can make a copy of this frame to create a new Macro frame)"
        n117 = call <vilib>:"Add State(s) to Queue__jki_lib_state_machine.vi"("State(s) in Front (\"\")"="Splash: Set Status >> Starting Instrument...\nSMO: Create Instrument\nSMO: Create Instrument UI\nEvents: Register\nSMO: Start Instrument\nSplash: Set Status >> Instrument Process Started...\nSplash: Set Status >> Starting User Interface...\nSMO: Start Instrument UI\nUI: Front Panel State >> Hide\nSMO: Show Instrument UI" ("State(s) in Front (\"\")"), "State(s) in (\"\")"=w320) -> ("States Out"=w319:string)  [unwired: 13 in]
      }
      frame "Macro: Stop SMOs" {
        # "Do not put any code in this frame.\n(It is a separator no-op. You can make a copy of this frame to create a new Macro frame)"
        n118 = call <vilib>:"Add State(s) to Queue__jki_lib_state_machine.vi"("State(s) in Front (\"\")"="//SMO: Hide Instrument UI\nSMO: Stop Instrument UI\nSMO: Stop Instrument\nSMO: Destroy Instrument UI\nSMO: Destroy Instrument" ("State(s) in Front (\"\")"), "State(s) in (\"\")"=w326) -> ("States Out"=w325:string)  [unwired: 13 in]
      }
      frame "Macro: Exit" {
        # "Exit Macro\n(This is called once, when the VI exits)"
        n119 = Unbundle By Name(w335) -> ("Core.Close Panel on Exit?"=w334:bool)
        n120 = Select(t="UI: Front Panel State >> Open", s=w334, f="") -> (s? t:f=w331:string)
        n121 = call <vilib>:"Add State(s) to Queue__jki_lib_state_machine.vi"("State(s) in Front (\"\")"="UI: Front Panel State >> Open\nUI: Exit", "State(s) in (\"\")"=w331, "State(s) at Back (\"\")"="Macro: Stop SMOs\nData: Cleanup\nEvents: Unregister\nExit") -> ("States Out"=w330:string)  [unwired: 12 in]
        n122 = call <vilib>:"Add State(s) to Queue__jki_lib_state_machine.vi"("State(s) in Front (\"\")"=w330, "State(s) in (\"\")"=w338) -> ("States Out"=w337:string)  [unwired: 13 in]
      }
      frame "---------- SMO ----------" {
        # "Do not put any code in this frame.\n(It is a separator no-op. You can make a copy of this frame to create a new Macro frame)"
        n123 = call <vilib>:"Add State(s) to Queue__jki_lib_state_machine.vi"("State(s) in (\"\")"=w343) -> ("States Out"=w342:string)  [unwired: 14 in]
      }
      frame "SMO: Create Instrument" {
        # "Do not put any code in this frame.\n(It is a separator no-op. You can make a copy of this frame to create a new Macro frame)"
        n124 = Unbundle By Name(w346) -> ("Instrument.Lockin"=w345:refnum<class "Instrument.Lockin.lvclass">)
        n125 = call-dynamic "Create Instrument SMO.vi"("error in (no error)"=w344, "Debug Mode? [F]"="Debug Mode?", "Configuration Window? [T]"=FALSE, "Instrument in"=w345) -> ("error out"=w347:errorcluster, "Instrument out"=w348:refnum<class "Instrument.Lockin.lvclass">)  [unwired: 6 in]
        n126 = Bundle By Name(cluster=w346, "Instrument.Lockin"=w348) -> (w351:T5)
        n127 = call <vilib>:"Add State(s) to Queue__jki_lib_state_machine.vi"("State(s) in (\"\")"=w354) -> ("States Out"=w353:string)  [unwired: 14 in]
      }
      frame "SMO: Start Instrument" {
        # "Do not put any code in this frame.\n(It is a separator no-op. You can make a copy of this frame to create a new Macro frame)"
        n128 = Unbundle By Name(w359) -> ("Instrument.Lockin"=w360:refnum<class "Instrument.Lockin.lvclass">)
        n129 = call <vilib>:"Start.vi"("error in (no error)"=w356, "SMO"=w360) -> ("error out"=w355:errorcluster, "SMO out"=w357:refnum<class "Instrument.Lockin.lvclass">)  [unwired: 8 in]
        n130 = Bundle By Name(cluster=w359, "Instrument.Lockin"=w357) -> (w358:T5)
        n131 = call <vilib>:"Add State(s) to Queue__jki_lib_state_machine.vi"("State(s) in (\"\")"=w363) -> ("States Out"=w362:string)  [unwired: 14 in]
      }
      frame "SMO: Stop Instrument" {
        # "Do not put any code in this frame.\n(It is a separator no-op. You can make a copy of this frame to create a new Macro frame)"
        n132 = Unbundle By Name(w370) -> ("Instrument.Lockin"=w365:refnum<class "Instrument.Lockin.lvclass">)
        n133 = call <vilib>:"GetState.vi"("error in (no error)"=w369, "SMO"=w365) -> ("error out"=w368:errorcluster, "SMO State"=w366:T1, "SMO out"=w364:refnum<class "Instrument.Lockin.lvclass">)  [unwired: 7 in]
        n134 = call <vilib>:"Clear Errors.vi"("error in (no error)"=w368) -> ("error out"=w367:errorcluster)  [unwired: 5 in, 1 out]
        n135 = case shown="\"Created\", \"Started\"" w366 {
          tunnel: [w375 w378] -> w371
          tunnel: w364 -> [_ w377]
          tunnel: w367 -> [w375 w376]
          frame Default {
          }
          frame "Created", "Started" {
            n136 = call <vilib>:"Stop.vi"("error in (no error)"=w376, "SMO"=w377) -> ("error out"=w378:errorcluster)  [unwired: 8 in, 1 out]
          }
        }
        n137 = call <vilib>:"Add State(s) to Queue__jki_lib_state_machine.vi"("State(s) in (\"\")"=w374) -> ("States Out"=w373:string)  [unwired: 14 in]
      }
      frame "SMO: Destroy Instrument" {
        # "Do not put any code in this frame.\n(It is a separator no-op. You can make a copy of this frame to create a new Macro frame)"
        n138 = Unbundle By Name(w386) -> ("Instrument.Lockin"=w384:refnum<class "Instrument.Lockin.lvclass">)
        n139 = call <vilib>:"GetState.vi"("error in (no error)"=w381, "SMO"=w384) -> ("error out"=w380:errorcluster, "SMO State"=w383:T1, "SMO out"=w379:refnum<class "Instrument.Lockin.lvclass">)  [unwired: 7 in]
        n140 = call <vilib>:"Clear Errors.vi"("error in (no error)"=w380) -> ("error out"=w382:errorcluster)  [unwired: 5 in, 1 out]
        n141 = case shown="Default" w383 {
          tunnel: [w390 w393] -> w385
          tunnel: w382 -> [w390 w392]
          tunnel: w379 -> [_ w391]
          frame Default {
          }
          frame "Stopped" {
            n142 = call <vilib>:"Destroy.vi"("error in (no error)"=w392, "SMO"=w391) -> ("error out"=w393:errorcluster)  [unwired: 9 in]
          }
        }
        n143 = call <vilib>:"Add State(s) to Queue__jki_lib_state_machine.vi"("State(s) in (\"\")"=w389) -> ("States Out"=w388:string)  [unwired: 14 in]
      }
      frame "SMO: Create Instrument UI" {
        # "Do not put any code in this frame.\n(It is a separator no-op. You can make a copy of this frame to create a new Macro frame)"
        n144 = Unbundle By Name(w400) -> ("Instrument UI.Lockin"=w394:refnum<class "Instrument UI.Lockin.lvclass">, "Instrument.Lockin"=w395:refnum<class "Instrument.Lockin.lvclass">)
        n145 = call <userlib>:"Create UI.vi"("error in (no error)"=w396, "Instrument in"=w395, "Instrument UI"=w394) -> ("error out"=w397:errorcluster, "Instrument UI out"=w398:refnum<class "Instrument UI.Lockin.lvclass">)  [unwired: 7 in]
        n146 = Bundle By Name(cluster=w400, "Instrument UI.Lockin"=w398) -> (w399:T5)
        n147 = call <vilib>:"Add State(s) to Queue__jki_lib_state_machine.vi"("State(s) in (\"\")"=w403) -> ("States Out"=w402:string)  [unwired: 14 in]
      }
      frame "SMO: Start Instrument UI" {
        # "Do not put any code in this frame.\n(It is a separator no-op. You can make a copy of this frame to create a new Macro frame)"
        n148 = Unbundle By Name(w407) -> ("Instrument UI.Lockin"=w406:refnum<class "Instrument UI.Lockin.lvclass">)
        n149 = call <vilib>:"Start.vi"("error in (no error)"=w405, "SMO"=w406) -> ("error out"=w404:errorcluster)  [unwired: 8 in, 1 out]
        n150 = call <vilib>:"Add State(s) to Queue__jki_lib_state_machine.vi"("State(s) in (\"\")"=w410) -> ("States Out"=w409:string)  [unwired: 14 in]
      }
      frame "SMO: Show Instrument UI" {
        # "Do not put any code in this frame.\n(It is a separator no-op. You can make a copy of this frame to create a new Macro frame)"
        n151 = Unbundle By Name(w418) -> ("Instrument UI.Lockin"=w416:refnum<class "Instrument UI.Lockin.lvclass">)
        n152 = call <vilib>:"GetState.vi"("error in (no error)"=w414, "SMO"=w416) -> ("error out"=w412:errorcluster, "SMO State"=w411:T1, "SMO out"=w415:refnum<class "Instrument UI.Lockin.lvclass">)  [unwired: 7 in]
        n153 = call <vilib>:"Clear Errors.vi"("error in (no error)"=w412) -> ("error out"=w413:errorcluster)  [unwired: 5 in, 1 out]
        n154 = case shown="\"Started\"" w411 {
          tunnel: [w422 w425] -> w417
          tunnel: w415 -> [_ w424]
          tunnel: w413 -> [w422 w423]
          frame Default {
          }
          frame "Started" {
            n155 = call <vilib>:"Show.vi"("error in (no error)"=w423, "SMO.UI"=w424) -> ("error out"=w425:errorcluster)  [unwired: 8 in, 1 out]
          }
        }
        n156 = call <vilib>:"Add State(s) to Queue__jki_lib_state_machine.vi"("State(s) in (\"\")"=w421) -> ("States Out"=w420:string)  [unwired: 14 in]
      }
      frame "SMO: Hide Instrument UI" {
        # "Do not put any code in this frame.\n(It is a separator no-op. You can make a copy of this frame to create a new Macro frame)"
        n157 = Unbundle By Name(w433) -> ("Instrument UI.Lockin"=w431:refnum<class "Instrument UI.Lockin.lvclass">)
        n158 = call <vilib>:"GetState.vi"("error in (no error)"=w429, "SMO"=w431) -> ("error out"=w427:errorcluster, "SMO State"=w426:T1, "SMO out"=w430:refnum<class "Instrument UI.Lockin.lvclass">)  [unwired: 7 in]
        n159 = call <vilib>:"Clear Errors.vi"("error in (no error)"=w427) -> ("error out"=w428:errorcluster)  [unwired: 5 in, 1 out]
        n160 = case shown="Default" w426 {
          tunnel: [w437 w440] -> w432
          tunnel: w430 -> [_ w439]
          tunnel: w428 -> [w437 w438]
          frame Default {
          }
          frame "Started" {
            n161 = call <vilib>:"Hide.vi"("error in (no error)"=w438, "SMO.UI"=w439) -> ("error out"=w440:errorcluster)  [unwired: 8 in, 1 out]
          }
        }
        n162 = call <vilib>:"Add State(s) to Queue__jki_lib_state_machine.vi"("State(s) in (\"\")"=w436) -> ("States Out"=w435:string)  [unwired: 14 in]
      }
      frame "SMO: Stop Instrument UI" {
        # "Do not put any code in this frame.\n(It is a separator no-op. You can make a copy of this frame to create a new Macro frame)"
        n163 = Unbundle By Name(w447) -> ("Instrument UI.Lockin"=w442:refnum<class "Instrument UI.Lockin.lvclass">)
        n164 = call <vilib>:"GetState.vi"("error in (no error)"=w446, "SMO"=w442) -> ("error out"=w445:errorcluster, "SMO State"=w443:T1, "SMO out"=w441:refnum<class "Instrument UI.Lockin.lvclass">)  [unwired: 7 in]
        n165 = call <vilib>:"Clear Errors.vi"("error in (no error)"=w445) -> ("error out"=w444:errorcluster)  [unwired: 5 in, 1 out]
        n166 = case shown="\"Created\", \"Started\"" w443 {
          tunnel: [w452 w455] -> w448
          tunnel: w441 -> [_ w454]
          tunnel: w444 -> [w452 w453]
          frame Default {
          }
          frame "Created", "Started" {
            n167 = call <vilib>:"Stop.vi"("error in (no error)"=w453, "SMO"=w454) -> ("error out"=w455:errorcluster)  [unwired: 8 in, 1 out]
          }
        }
        n168 = call <vilib>:"Add State(s) to Queue__jki_lib_state_machine.vi"("State(s) in (\"\")"=w451) -> ("States Out"=w450:string)  [unwired: 14 in]
      }
      frame "SMO: Destroy Instrument UI" {
        # "Do not put any code in this frame.\n(It is a separator no-op. You can make a copy of this frame to create a new Macro frame)"
        n169 = Unbundle By Name(w462) -> ("Instrument UI.Lockin"=w461:refnum<class "Instrument UI.Lockin.lvclass">)
        n170 = call <vilib>:"GetState.vi"("error in (no error)"=w459, "SMO"=w461) -> ("error out"=w458:errorcluster, "SMO State"=w456:T1, "SMO out"=w460:refnum<class "Instrument UI.Lockin.lvclass">)  [unwired: 7 in]
        n171 = call <vilib>:"Clear Errors.vi"("error in (no error)"=w458) -> ("error out"=w457:errorcluster)  [unwired: 5 in, 1 out]
        n172 = case shown="\"Stopped\"" w456 {
          tunnel: w457 -> [w467 w470]
          tunnel: [w467 w469] -> w463
          tunnel: w460 -> [_ w468]
          frame Default {
          }
          frame "Stopped" {
            n173 = call <vilib>:"Destroy.vi"("error in (no error)"=w470, "SMO"=w468) -> ("error out"=w469:errorcluster)  [unwired: 9 in]
          }
        }
        n174 = call <vilib>:"Add State(s) to Queue__jki_lib_state_machine.vi"("State(s) in (\"\")"=w466) -> ("States Out"=w465:string)  [unwired: 14 in]
      }
      frame "---------- Splash ----------" {
        # "Template Separator\n(You can make a copy of, or modify, this frame)"
        n175 = call <vilib>:"Add State(s) to Queue__jki_lib_state_machine.vi"("State(s) in (\"\")"=w475) -> ("States Out"=w474:string)  [unwired: 14 in]
      }
      frame "Splash: Set Status" {
        # "Your code here.\n(You can make a copy of, or modify, this frame)"
        n176 = property on="Splash Status" class="Str"(error in=w478, "Value"=w479) -> (error out=w477:errorcluster)  [unwired: 1 in, 1 out]
        n177 = call <vilib>:"Add State(s) to Queue__jki_lib_state_machine.vi"("State(s) in (\"\")"=w482) -> ("States Out"=w481:string)  [unwired: 14 in]
      }
      frame "Splash: 2" {
        # "Your code here.\n(You can make a copy of, or modify, this frame)"
        n178 = call <vilib>:"Add State(s) to Queue__jki_lib_state_machine.vi"("State(s) in (\"\")"=w487) -> ("States Out"=w486:string)  [unwired: 14 in]
      }
    }
  }
  "error out" <- w1
